vi "test_libssh2_session_supported_algs.vi"() -> ()   [LabVIEW 2013, in "libssh2_integration_tests.lvlib"]
uses:
  libssh2_integration_tests.lvlib
  libssh2/libssh2_method_type.ctl
  <vilib>/addons/_JKI Toolkits/Caraya/classes/Test/Test.lvclass
  libssh2/libssh2.lvlib
  Assert Extensions/Assert Extensions.lvclass
panel:
  out "error out":errorcluster
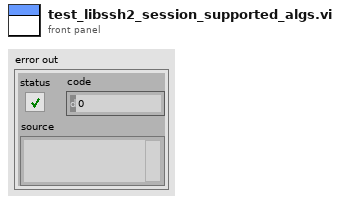
[diagram p1: front panel]
types:
  T1 = typedef "libssh2.lvlib/libssh2_method_type.ctl" = enum16{"LIBSSH2_METHOD_KEX", "LIBSSH2_METHOD_HOSTKEY", "LIBSSH2_METHOD_CRYPT_CS", "LIBSSH2_METHOD_CRYPT_SC", "LIBSSH2_METHOD_MAC_CS", "LIBSSH2_METHOD_MAC_SC", "LIBSSH2_METHOD_COMP_CS", "LIBSSH2_METHOD_COMP_SC", "LIBSSH2_METHOD_LANG_CS", "LIBSSH2_METHOD_LANG_SC", "LIBSSH2_METHOD_SIGN_ALGO"}
  T2 = typedef "libssh2.lvlib/Session Refnum.ctl" = refnum<k1>
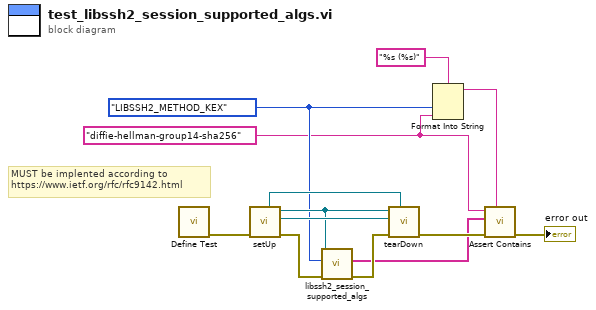
[diagram p0: block diagram]
diagram:
  w2 = "diffie-hellman-group14-sha256" ("string")
  w4 = libssh2_method_type."LIBSSH2_METHOD_KEX" ("method_type")
  # "MUST be implented according to\nhttps://www.ietf.org/rfc/rfc9142.html"
  n1 = call <vilib>:"Define Test.vi"() -> ("error out"=w13:errorcluster)  [unwired: 10 in, 1 out]
  n2 = call "setUp.vi"("error in (no error)"=w13) -> ("error out"=w8:errorcluster, "connection ID"=w12:refnum<k5>, "session"=w10:T2, "fixture"=w11:refnum<class "Server Fixture.lvclass">)  [unwired: 7 in]
  n3 = call "libssh2_session_supported_algs.vi"("error in (no error)"=w8, "method_type"=w4, "session"=w10) -> ("error out"=w9:errorcluster, "algs"=w3:string[])  [unwired: 7 in]
  n4 = call "tearDown.vi"("fixture"=w11, "error in (no error)"=w9, "connection ID"=w12, "session"=w10) -> ("error out"=w7:errorcluster)  [unwired: 7 in]
  n5 = Format Into String(format string="%s (%s)", w4, w2) -> (resulting string=w6:string)  [unwired: 2 in, 1 out]
  n6 = call "Assert Contains.vi"("Label"=w6, "error in (no error)"=w7, "Array"=w3, "Item"=w2) -> ("error out"=→"error out":errorcluster)  [unwired: 7 in]
